vi "svx_Build Orbit and Timebase Data (N Ch - M Orders).vi"(0 "order data":dbl[][][](array[numeric]), 1 "magnitudes info":T1[](array[typedef]) {"x-axis units" items=["Time (s)"=0, "Frequency-CB (Hz)"=1, "Frequency-CPB (Hz)"=1248, "Frequency-Arbitrary (Hz)"=2357, "Quefrency (s)"=2, "Revolutions (rev)"=3, "Order"=4, "Speed (RPM)"=11, "Speed (rad/s)"=21, "Index"=65535]; "weighting filter" items=["Linear", "A-weighting", "B-weighting", "C-weighting", "ITU-R 468-4", "Dolby", "CCITT", "C-message", "Wb", "Wc", "Wd", "We", "Wf", "Wh", "Wj", "Wk", "Wm", "AES17 20 kHz lowpass", "AES17 40 kHz lowpass", "AES17 20 kHz highpass", "AES17 40 kHz highpass"]; "dB reference [EU]" format="%.2f"; "engineering units" items=["custom..."=0, "V"=1, "A"=21, "C"=30, "pC"=31, "s"=32, "-"=29, "Pa"=2, "N"=20, "g"=3, "m/s^2"=4, "m/s"=5, "m"=6, "mm/s"=12, "mm"=13, "micron/s"=14, "micron"=15, "in/s^2"=7, "in/s"=8, "in"=9, "mil/s"=10, "mil"=11, "rad/s^2"=16, "rad/s"=17, "rad"=18, "deg/s^2"=26, "deg/s"=27, "deg"=28, "RPM"=22, "cycle/s^2"=23, "Hz"=24, "cycle"=25, "strain"=19]; "spectral info"."window" items=["None "=0, "Hanning"=1, "Hamming"=2, "Blackman-Harris"=3, "Exact Blackman"=4, "Blackman"=5, "Flat Top"=6, "4 Term B-Harris "=7, "7 Term B-Harris"=8, "Low Sidelobe"=9, "Force - Exponential"=10, "Gaussian"=62]}, 5 "interpolated pulse positions[s]":dbl[](array[numeric]) format="%.2f", 7 "actual samples/rev":dbl=1.0 format="%.2f", 9 "orders":dbl[](array[numeric]), 11 "error in (no error)":errorcluster, 12 "channel properties":T7[](array[typedef]) {"probe angle [deg]" max=360; "direction" items=["CCW", "CW"]}, 14 "pair index":cluster{"index 1":i32, "index 2":i32}[](array[cluster])) -> (4 "orbit/timebase plot":T8(array[cluster]), 15 "error out":errorcluster)   [LabVIEW 2017]
uses:
  <vilib>/addons/Sound and Vibration/Order Analysis/Data Presentation/SubVIs/OAT MCM Channel Property.ctl
  <vilib>/addons/_NISVFA/_Shared subVIs/Controls/svc_Spectrum Info.ctl
  <vilib>/addons/_NISVFA/_Shared subVIs/Controls/svc_X-Axis Units.ctl
  <vilib>/addons/_NISVFA/_Shared subVIs/Controls/svc_Spectrum Type.ctl
  <vilib>/addons/_NISVFA/_Shared subVIs/Controls/svc_Engineering Units Text Ring.ctl
  <vilib>/addons/_NISVFA/_Shared subVIs/Controls/svc_Weighting Filter Text Ring.ctl
  <vilib>/addons/_NISVFA/_Shared subVIs/Controls/svc_Complimentary Spectrum Units.ctl
  <vilib>/addons/Sound and Vibration/Order Analysis/Misc/SVMS Attribute.ctl
  <vilib>/addons/_NISVFA/_Shared subVIs/Controls/NI Channel Properties.ctl
  <vilib>/addons/_NISVFA/_Shared subVIs/Common/svc_Get Weighting Enum and Labels.vi
  <vilib>/addons/_NISVFA/_Shared subVIs/Common/svc_Unit Label Lexical Class.vi
  <vilib>/addons/_NISVFA/_Shared subVIs/Common/svc_Engineering Units to Unit Label.vi
  <vilib>/addons/_NISVFA/_Shared subVIs/Common/svc_Format Value (DBL).vi
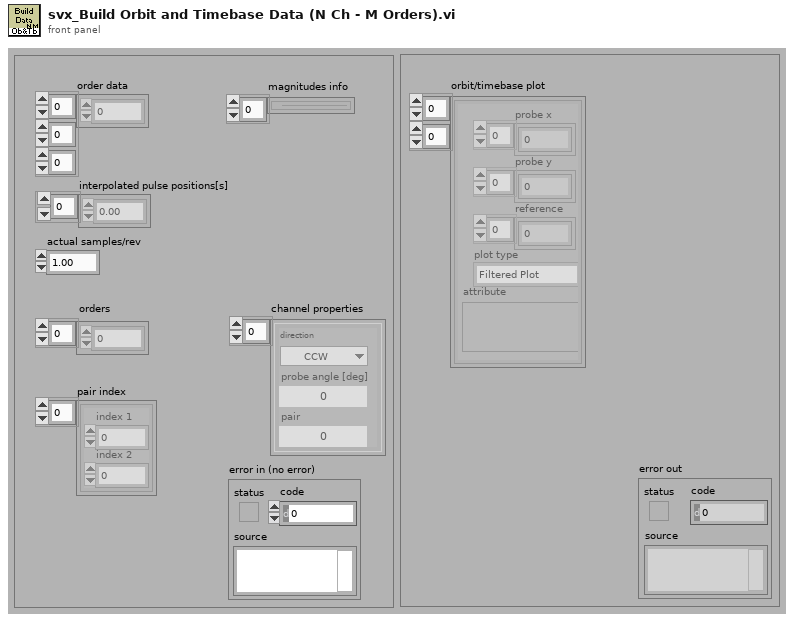
[diagram p1: front panel]
types:
  T1 = typedef "svc_Spectrum Info.ctl" = cluster{"channel name":string, "description":string, "x-axis units":T2, "spectral info":cluster{"spectrum type":T3, "linear/dB":enum16{"linear", "dB"}, "window":u16, "window size":i32, "FFT size":i32}, "engineering units":T4, "custom label":string, "dB reference [EU]":dbl, "peak units":enum16{"rms", "peak", "peak-peak"}, "weighting filter":T5, "spectral density?":bool, "unit label":string, "spectrum skewed?":bool, "complimentary spectrum units":T6}
  T2 = typedef "svc_X-Axis Units.ctl" = u16
  T3 = typedef "svc_Spectrum Type.ctl" = enum16{"FFT Spectrum [complex]", "Amplitude [Magnitude]", "Power [Magnitude^2]", "Cross Spectrum [complex]", "Frequency Response [Complex]"}
  T4 = typedef "svc_Engineering Units Text Ring.ctl" = u16
  T5 = typedef "svc_Weighting Filter Text Ring.ctl" = u16
  T6 = typedef "svc_Complimentary Spectrum Units.ctl" = enum16{"none", "radians", "degrees", "cycles", "imaginary"}
  T7 = typedef "OAT MCM Channel Property.ctl" = cluster{"direction":u16, "probe angle [deg]":u16, "pair":u16}
  T8 = cluster{"probe x":dbl[], "probe y":dbl[], "reference":dbl[], "plot type":enum16{"Filtered Plot", "Unfiltered Plot"}, "attribute":variant}[][]
  T9 = cluster{"X":dbl[], "Y":dbl[], "reference":dbl[], "plot type":enum16{"Filtered Plot", "Unfiltered Plot"}, "attribute":variant}
  T10 = typedef "NI Channel Properties.ctl" = u16
  T11 = typedef "SVMS Attribute.ctl" = u16
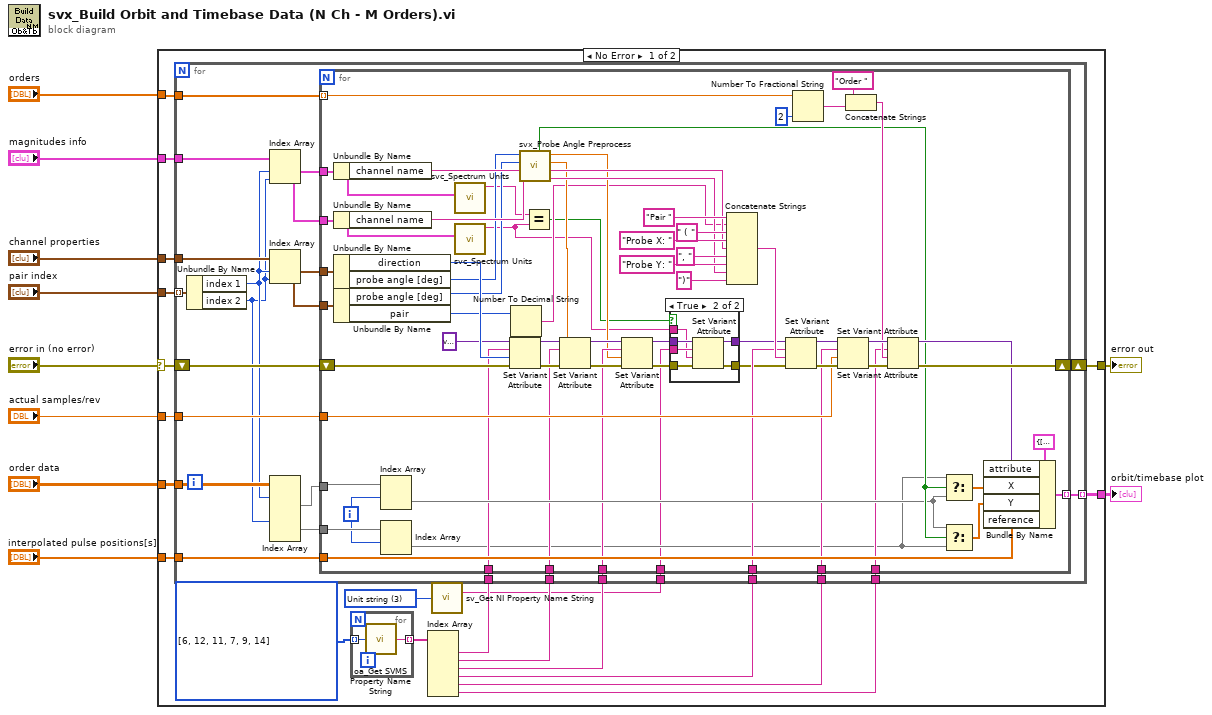
[diagram p0: block diagram]
diagram:
  n1 = case shown="No Error" "error in (no error)" {
    selector: "error in (no error)" -> [w28 w131]
    tunnel: "channel properties" -> [w30 _]
    tunnel: "order data" -> [w29 _]
    tunnel: [w25 w131] -> w8
    tunnel: "actual samples/rev" -> [w27 _]
    tunnel: "orders" -> [w26 _]
    tunnel: "interpolated pulse positions[s]" -> [w24 _]
    tunnel: "magnitudes info" -> [w23 _]
    tunnel: "pair index" -> [w22 _]
    tunnel: [w21 _] -> w1
    frame No Error {
      w12 = T10 3 items=["Channel name", "Channel description", "Axis label", "Unit string", "Waveform X-axis label", "Waveform X-axis unit string", "x0", "dx", "Number of samples", "X channel", "Filter settled", "dB reference", "Window", "Window parameter", "Window size", "FFT size", "Peak units", "Spectrum type", "Magnitude scale", "Spectral density", "Sensor sensitivity (mV/EU)", "X-axis dimension", "LabVIEW datatype", "Function type", "Function subtype", "X values", "Independent channel", "Column index", "Collection name", "Collection ID", "X Columns", "Phase unwrapped", "Sensor type", "Sensor maximum", "Averaging mode"] ("property")
      w20 = T11[] [6, 12, 11, 7, 9, 14] items=["Pulse / Revolution", "Slope", "Threshold", "Hysteresis", "Order", "Reference Label", "Rotation Direction", "Pair String", "Polar Plot Type", "Sample Per Revolution", "Probe Angle", "Probe Angle X", "Probe Angle Y", "X Axis Unit", "OTB Plot Type"]
      n2 = for {
        tunnel: w20 -> [w32] mode=indexing
        tunnel: [w31] -> w19 mode=indexing
        n3 = call <vilib>:"oa_Get SVMS Property Name String.vi"("attribute"=w32) -> ("attribute name"=w31:string)  [unwired: 4 in]
      }
      n4 = Index Array(array=w19) -> (element #1=w18:string, element #2=w17:string, element #3=w16:string, element #4=w15:string, element #5=w14:string, element #6=w13:string)  [unwired: 6 in]
      n5 = call <vilib>:"sv_Get NI Property Name String.vi"("property"=w12) -> ("TDMS property name"=w11:string)  [unwired: 13 in, 1 out]
      n6 = for {
        shift-right: [w57] -> w25
        shift-left: w28 -> [w50]
        tunnel: w27 -> [w56]
        tunnel: w26 -> [w55]
        tunnel: w24 -> [w54]
        tunnel: w29 -> [w49]
        tunnel: w22 -> [w48] mode=indexing
        tunnel: w30 -> [w53]
        tunnel: w23 -> [w46]
        tunnel: [w40] -> w21 mode=indexing
        tunnel: w18 -> [w39]
        tunnel: w17 -> [w38]
        tunnel: w16 -> [w37]
        tunnel: w15 -> [w36]
        tunnel: w14 -> [w35]
        tunnel: w13 -> [w34]
        tunnel: w11 -> [w33]
        n7 = Unbundle By Name(w48) -> ("index 1"=w45:i32, "index 2"=w44:i32)
        n8 = Index Array(array=w46, index #1=w45, index #2=w44) -> (element #1=w43:T1, element #2=w41:T1)
        n9 = Index Array(array=w53, index #1=w45, index #2=w44) -> (element #1=w52:T7, element #2=w51:T7)
        n10 = Index Array(array=w49, index (dim 0) #1=w45, index (dim 0) #2=w44) -> (element #1=w47:dbl[][], element #2=w42:dbl[][])  [unwired: 4 in]
        n11 = for {
          tunnel: w52 -> [w122]
          tunnel: w51 -> [w121]
          shift-right: [w106] -> w57
          shift-left: w50 -> [w115]
          tunnel: w47 -> [w98]
          tunnel: w42 -> [w97]
          tunnel: [w110] -> w40 mode=indexing
          tunnel: w56 -> [w102]
          tunnel: w55 -> [w99] mode=indexing
          tunnel: w54 -> [w95]
          tunnel: w43 -> [w66]
          tunnel: w41 -> [w65]
          tunnel: w39 -> [w77]
          tunnel: w38 -> [w76]
          tunnel: w37 -> [w75]
          tunnel: w36 -> [w74]
          tunnel: w35 -> [w73]
          tunnel: w34 -> [w72]
          tunnel: w33 -> [w62]
          i -> [w96]
          n12 = Unbundle By Name(w66) -> ("channel name"=w87:string)
          n13 = Unbundle By Name(w65) -> ("channel name"=w86:string)
          n14 = Unbundle By Name(w122) -> ("direction"=w116:u16, "probe angle [deg]"=w85:u16)
          n15 = Unbundle By Name(w121) -> ("probe angle [deg]"=w84:u16, "pair"=w111:u16)
          n16 = Index Array(array=w98, index (row)=w96) -> (element=w79:dbl[])  [unwired: 1 in]
          n17 = Index Array(array=w97, index (row)=w96) -> (element=w71:dbl[])  [unwired: 1 in]
          n18 = call <vilib>:"svc_Spectrum Units.vi"("spectrum info in"=w66) -> ("unit label"=w67:string)  [unwired: 3 in, 3 out]
          n19 = call <vilib>:"svc_Spectrum Units.vi"("spectrum info in"=w65) -> ("unit label"=w60:string)  [unwired: 3 in, 3 out]
          n20 = Set Variant Attribute(Variant=variant ("variant"), name=w77, value=w116, error in=w115) -> (Variant out=w120:variant, error out=w119:errorcluster)  [unwired: 1 out]
          n21 = Number To Decimal String(number=w111) -> (decimal integer string=w68:string)  [unwired: 1 in]
          n22 = call <vilib>:"svx_Probe Angle Preprocess.vi"("channel name Y"=w86, "channel name X"=w87, "Y"=w84, "X"=w85) -> ("actual Y"=w82:string, "actual X"=w83:string, "Y"=w69:dbl, "X"=w70:dbl, "switched?"=w80:bool)  [unwired: 3 in]
          n23 = Equal?(x=w67, y=w60) -> (x = y?=w61:bool)
          n24 = Set Variant Attribute(Variant=w120, name=w76, value=w69, error in=w119) -> (Variant out=w117:variant, error out=w118:errorcluster)  [unwired: 1 out]
          n25 = Set Variant Attribute(Variant=w117, name=w75, value=w70, error in=w118) -> (Variant out=w64:variant, error out=w63:errorcluster)  [unwired: 1 out]
          n26 = case shown="True" w61 {
            tunnel: w63 -> [w123 w130]
            tunnel: w64 -> [w124 w129]
            tunnel: [w123 w128] -> w58
            tunnel: [w124 w127] -> w59
            tunnel: w62 -> [_ w126]
            tunnel: w60 -> [_ w125]
            frame False {
            }
            frame True {
              n27 = Set Variant Attribute(Variant=w129, name=w126, value=w125, error in=w130) -> (Variant out=w127:variant, error out=w128:errorcluster)  [unwired: 1 out]
            }
          }
          n28 = Concatenate Strings("Pair " ("string"), w68, " ( " ("string"), "Probe X: " ("string"), w83, ", " ("string"), "Probe Y: " ("string"), w82, ")" ("string")) -> (w91:string)
          n29 = Set Variant Attribute(Variant=w59, name=w74, value=w91, error in=w58) -> (Variant out=w112:variant, error out=w113:errorcluster)  [unwired: 1 out]
          n30 = Number To Fractional String(number=w99, precision (6)=i16 2) -> (F-format string=w105:string)  [unwired: 2 in]
          n31 = Set Variant Attribute(Variant=w112, name=w73, value=w102, error in=w113) -> (Variant out=w108:variant, error out=w109:errorcluster)  [unwired: 1 out]
          n32 = Concatenate Strings("Order " ("string"), w105) -> (w103:string)
          n33 = Set Variant Attribute(Variant=w108, name=w72, value=w103, error in=w109) -> (Variant out=w100:variant, error out=w106:errorcluster)  [unwired: 1 out]
          n34 = Select(t=w71, s=w80, f=w79) -> (s? t:f=w81:dbl[])
          n35 = Select(t=w79, s=w80, f=w71) -> (s? t:f=w78:dbl[])
          n36 = Bundle By Name(cluster=T9 {"X"=[], "Y"=[], "reference"=[], "plot type"=enum."Filtered Plot", "attribute"=variant} ("orbit plot 2"), "attribute"=w100, "X"=w81, "Y"=w78, "reference"=w95) -> (w110:T9)
        }
      }
    }
    frame Error {
    }
  }
  "orbit/timebase plot" <- w1
  "error out" <- w8
